vi "Wilt Dryer Cluster Arrays ReadWrite.vi"(0 "Array Label":string(combo)="Aisle1", 1 "Write?":bool, 5 "configuration file path":path=path "C:/data/Wilt Backup.ini", 7 "Array Dryers In":T1[](array[typedef]) {"Night Cycle Count" format="%04d"; "Dryer Details"."Stop Dryer" items=["NO", "YES"]; "Dryer Details"."24 Hour Water Injection" items=["NO", "YES"]; "Dryer Details"."Run w/o Newfi" items=["NO", "YES"]; "Day Cycle Count" format="%04d"}, 11 "error in (no error)":errorcluster) -> (8 "Array Dryers Out":T1[](array[typedef]) {"Night Cycle Count" format="%04d"; "Dryer Details"."Stop Dryer" items=["NO", "YES"]; "Dryer Details"."24 Hour Water Injection" items=["NO", "YES"]; "Dryer Details"."Run w/o Newfi" items=["NO", "YES"]; "Day Cycle Count" format="%04d"}, 15 "error out":errorcluster)   [LabVIEW 2012]
uses:
  <vilib>/Utility/VariantDataType/Type.ctl
  Dryer.ctl
  Dryer Details.ctl
  <vilib>/Utility/config.llb/Write Key (Double).vi
  <vilib>/Utility/config.llb/Write Key (String).vi
  <vilib>/Utility/config.llb/Write Key (Path).vi
  <vilib>/Utility/config.llb/Write Key (I32).vi
  <vilib>/Utility/config.llb/Write Key (U32).vi
  <vilib>/Utility/config.llb/Write Key (Boolean).vi
  <vilib>/Utility/config.llb/Read Key (Double).vi
  <vilib>/Utility/config.llb/Read Key (String).vi
  <vilib>/Utility/config.llb/Read Key (Path).vi
  <vilib>/Utility/config.llb/Read Key (I32).vi
  <vilib>/Utility/config.llb/Read Key (U32).vi
  <vilib>/Utility/config.llb/Read Key (Boolean).vi
  <vilib>/Utility/config.llb/NI_LVConfig.lvlib
  <vilib>/Utility/VariantDataType/VariantType.lvlib
panel:
  out "Label.Text 2":string
  out "Local Control?":bool
  in  "Array Dryers Display":T1[](array[typedef]) {"Night Cycle Count" format="%04d"; "Dryer Details"."Stop Dryer" items=["NO", "YES"]; "Dryer Details"."24 Hour Water Injection" items=["NO", "YES"]; "Dryer Details"."Run w/o Newfi" items=["NO", "YES"]; "Day Cycle Count" format="%04d"}
  out "value":string
  in  "Dryer Variable":T1 {"Night Cycle Count" format="%04d"; "Dryer Details"."Stop Dryer" items=["NO", "YES"]; "Dryer Details"."24 Hour Water Injection" items=["NO", "YES"]; "Dryer Details"."Run w/o Newfi" items=["NO", "YES"]; "Day Cycle Count" format="%04d"}
  out "String array out":string="[1,23-2-3]\n[4-3,22-2]\n[3-4,01-8]\n[0-7-6,66]"
  out "Label.Text":string
  out "Type Enum":T3
  # "D"
  # "N"
  # "D"
  # "N"
  # "D"
  # "N"
  # "D"
  # "N"
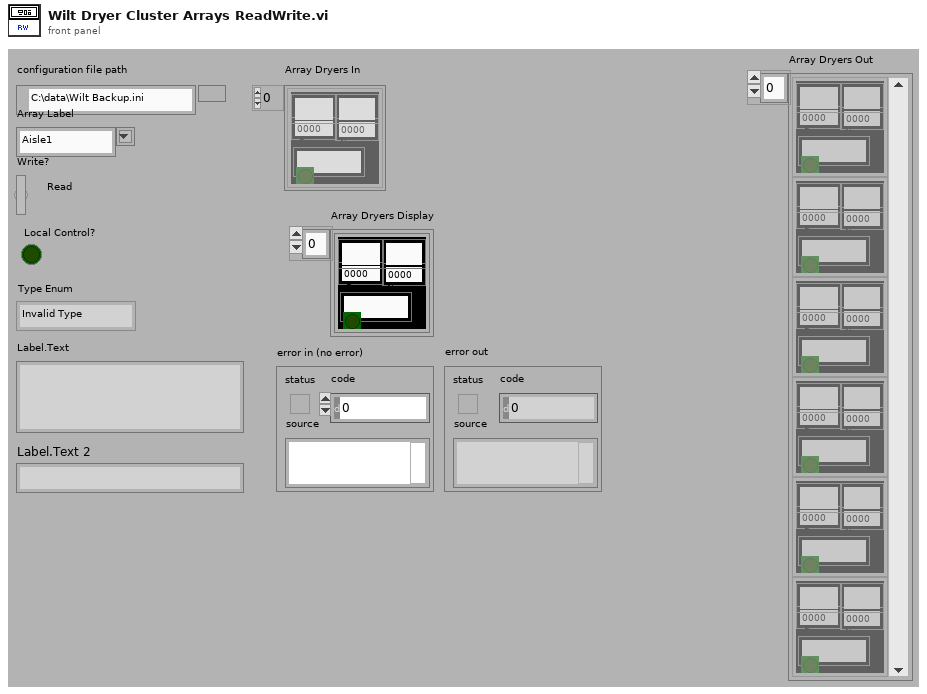
[diagram p1: front panel]
types:
  T1 = typedef "Dryer.ctl" = cluster{"Lab ID":string, "Day Cycle Count":i32, "Station Label":string, "Dryer Details":T2, "Sample Record ":string[], "Hist Record ":string[][], "Status Color":u32, "Boolean":bool, "Com Port":u8, "Bad Com Count":i32, "Current Run Start Time":dbl, "Night Cycle Count":i32, "Station Index":i32, "Cycle Index":string, "Audit Alert":bool}
  T2 = typedef "Dryer Details.ctl" = cluster{"Station":string, "Cycle Count Day":string, "Status":string, "Debug ASCII":string, "Notes":string, "Lab ID":string, "Total Time On":string, "TR Number":string, "Cycle Count Night":string, "Time On Day":string, "Time On Night":string, "Run w/o Newfi":i32, "24 Hour Water Injection":i32, "Stop Dryer":i32}
  T3 = typedef "VariantType.lvlib/Type.ctl" = enum8{"Invalid Type", "Void", "I8", "I16", "I32", "I64", "U8", "U16", "U32", "U64", "Single Float", "Double Float", "Extended Float", "Single Complex", "Double Complex", "Extended Complex", "Enum U8", "Enum U16", "Enum U32", "Enum U64", "Single Float With Unit", "Double Float With Unit", "Extended Float With Unit", "Single Complex with Unit", "Double Complex with Unit", "Extended Complex with Unit", "Boolean", "String", "Path", "Picture", "Tag", "Array", "Cluster", "Variant", "LV Variant", "Waveform", "Timestamp", "Digital Waveform", "Digital Data", "ExpressData", "Refnum", "External Data", "VI", "Poly VI", "LabVIEW Class Instance", "Fixed Point"}
  T4 = typedef "NI_LVConfig.lvlib/Config Data RefNum.ctl" = refnum<k1>
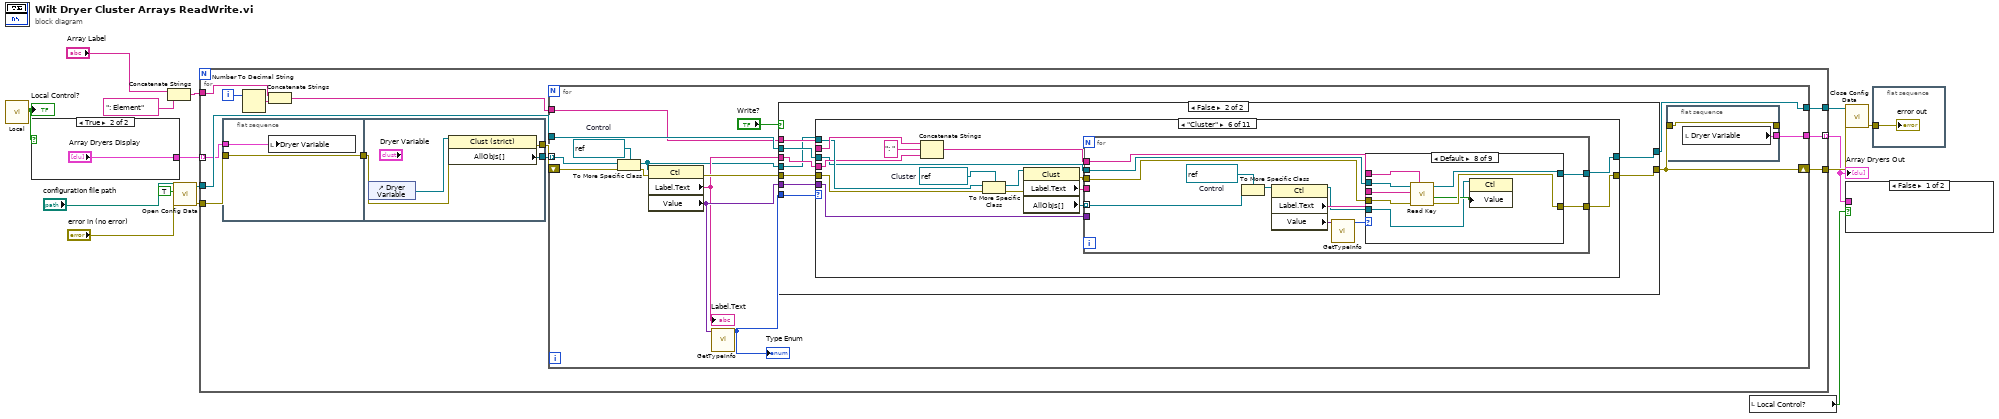
[diagram p0: block diagram]
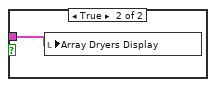
[diagram p2: hidden frame]
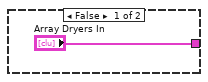
[diagram p3: hidden frame]
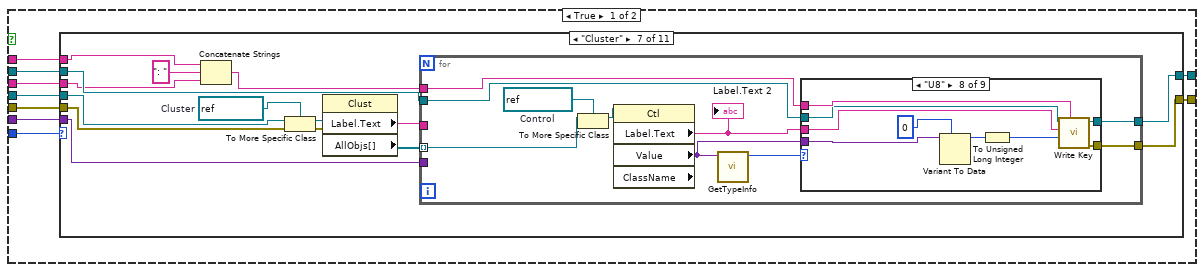
[diagram p4: hidden frame]
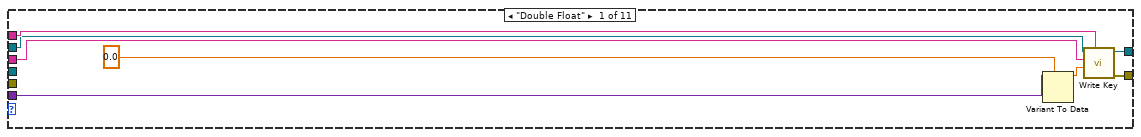
[diagram p5: hidden frame]
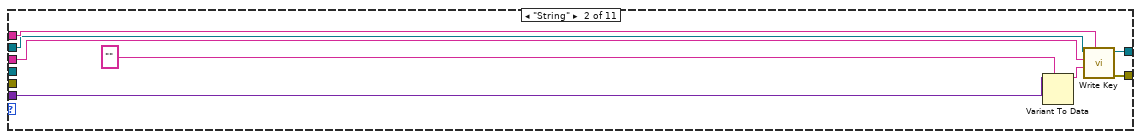
[diagram p6: hidden frame]
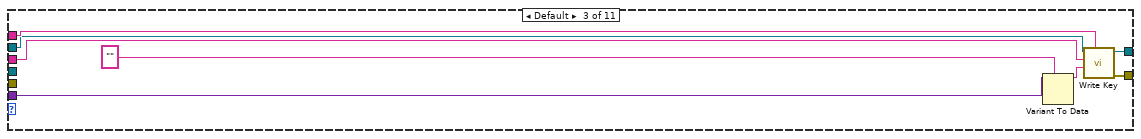
[diagram p7: hidden frame]
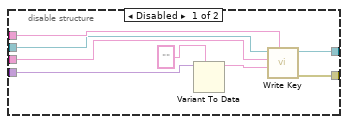
[diagram p9: hidden frame]
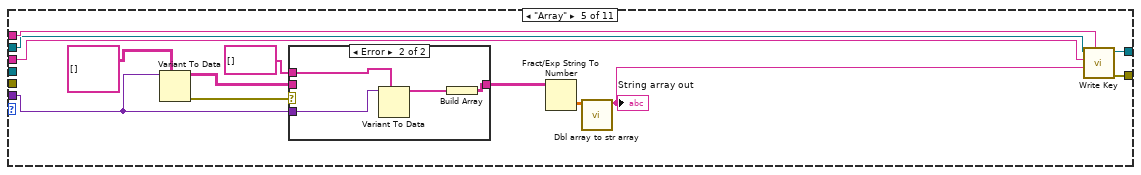
[diagram p10: hidden frame]
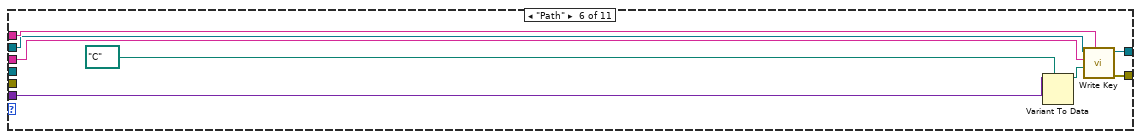
[diagram p12: hidden frame]
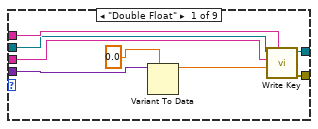
[diagram p13: hidden frame]
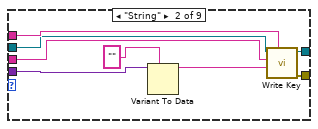
[diagram p14: hidden frame]
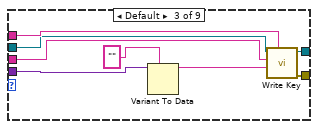
[diagram p15: hidden frame]
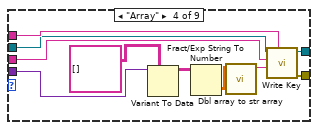
[diagram p16: hidden frame]
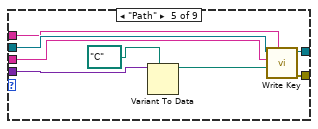
[diagram p17: hidden frame]
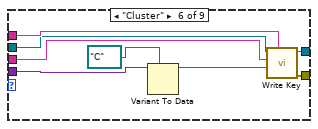
[diagram p18: hidden frame]
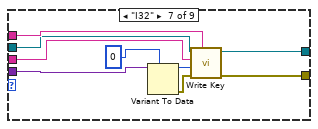
[diagram p19: hidden frame]
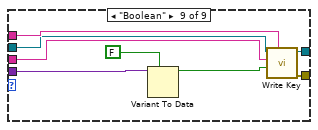
[diagram p20: hidden frame]
diagram:
  n1 = call "Local.vi"() -> ("Local?"=w1:bool)  [unwired: 11 in]
  "Local Control?" <- w1
  n2 = case shown="True" w1 {
    tunnel: ["Array Dryers In" "Array Dryers Display"] -> w3
    frame False {
    }
    frame True {
    }
  }
  n3 = Concatenate Strings("Array Label", ": Element" ("string")) -> (w8:string)
  n4 = call <vilib>:"Open Config Data.vi"("error in (no error)"="error in (no error)", "create file if necessary (T)"=TRUE, "configuration file path"="configuration file path") -> ("error out"=w11:errorcluster, "refnum"=w13:T4)  [unwired: 6 in, 1 out]
  n5 = for {
    tunnel: w11 -> [w29]
    tunnel: w3 -> [w25] mode=indexing
    tunnel: w13 -> [w27]
    tunnel: w8 -> [w23]
    tunnel: [w20] -> w6
    tunnel: [w19] -> w5
    tunnel: [w18] -> w4 mode=indexing
    i -> [w21]
    n6 = flat-sequence {
      tunnel: w29 -> [w32]
      tunnel: [w32] -> w26
      tunnel: w25 -> [w31]
      tunnel: [w36] -> w30
      tunnel: [w34] -> w28
      tunnel: w26 -> [w35]
      frame #0 {
        n7 = local write "Dryer Variable"(w31) -> ()
      }
      frame #1 {
        n8 = control-ref of="Dryer Variable"() -> (w33:refnum<vi>)
        n9 = property class="Clust (strict)"(reference=w33, error in=w35) -> (error out=w34:errorcluster, "AllObjs[]"=w36:refnum<vi>[])  [unwired: 1 out]
      }
    }
    n10 = Number To Decimal String(number=w21) -> (decimal integer string=w24:string)  [unwired: 1 in]
    n11 = Concatenate Strings(w23, w24) -> (w22:string)
    n12 = for {
      tunnel: w30 -> [w51] mode=indexing
      tunnel: w27 -> [w49]
      tunnel: [w48] -> w19
      shift-right: [w39] -> w20
      shift-left: w28 -> [w47]
      tunnel: w22 -> [w40]
      tunnel: [w38] -> w18
      w50 = refnum<vi> refnum  # Control
      n13 = To More Specific Class(target class=w50, reference=w51, error in=w47) -> (specific class reference=w37:refnum<vi>, error out=w42:errorcluster)
      n14 = property class="Ctl"(reference=w37, error in=w42) -> (error out=w43:errorcluster, "Label.Text"=w41:string, "Value"=w44:variant)  [unwired: 1 out]
      "Label.Text" <- w41
      n15 = call <vilib>:"GetTypeInfo.vi"("Variant"=w44) -> ("Type Enum"=w45:T3)  [unwired: 6 in, 4 out]
      "Type Enum" <- w45
      n16 = case shown="False" "Write?" {
        tunnel: w40 -> [w62 w269]
        tunnel: w41 -> [w61 w268]
        tunnel: w44 -> [w60 w261]
        tunnel: w49 -> [w59 w267]
        tunnel: [w58 w266] -> w39
        tunnel: [w57 w265] -> w48
        tunnel: w37 -> [w54 w264]
        tunnel: w45 -> [w56 w263]
        tunnel: w43 -> [w55 w262]
        frame True {
          n17 = case shown="\"Cluster\"" w56 {
            tunnel: w62 -> [w70 w78 w86 w92 w113 w126 w129 w235 w243 w252 w260]
            tunnel: w61 -> [w69 w77 w85 w91 w112 w125 w128 w234 w242 w251 w259]
            tunnel: w60 -> [w68 w76 w84 w90 w102 w124 w137 w233 w241 w250 w258]
            tunnel: w59 -> [w67 w75 w83 w89 w111 w123 w131 w232 w240 w249 w257]
            tunnel: [w66 w74 w82 w88 w110 w122 w135 w231 w239 w248 w256] -> w58
            tunnel: [w65 w73 w81 w87 w109 w121 w136 w230 w238 w247 w255] -> w57
            tunnel: w55 -> [_ _ _ _ _ _ w138 _ _ _ _]
            tunnel: w54 -> [_ _ _ _ _ _ w133 _ _ _ _]
            frame "Double Float" {
              n18 = Variant To Data(type=0.0, Variant=w68) -> (data=w64:dbl)  [unwired: 1 in, 1 out]
              n19 = call-poly <vilib>:"Write Key.vi"("section"=w70, "value"=w64, "key"=w69, "refnum"=w67) -> ("error out"=w66:errorcluster, "refnum out"=w65:T4)  [unwired: 5 in, 1 out]
            }
            frame "String" {
              n20 = Variant To Data(type="" ("Label.Text"), Variant=w76) -> (data=w72:string)  [unwired: 1 in, 1 out]
              n21 = call-poly <vilib>:"Write Key.vi"("section"=w78, "value"=w72, "key"=w77, "refnum"=w75) -> ("error out"=w74:errorcluster, "refnum out"=w73:T4)  [unwired: 5 in, 1 out]
            }
            frame Default {
              n22 = Variant To Data(type="" ("Label.Text"), Variant=w84) -> (data=w80:string)  [unwired: 1 in, 1 out]
              n23 = call-poly <vilib>:"Write Key.vi"("section"=w86, "value"=w80, "key"=w85, "refnum"=w83) -> ("error out"=w82:errorcluster, "refnum out"=w81:T4)  [unwired: 5 in, 1 out]
            }
            frame "Void" {
              n24 = disable-structure shown="Enabled" {
                disable-tunnel: w92 -> [w100 _]
                disable-tunnel: w91 -> [w99 _]
                disable-tunnel: w90 -> [w98 _]
                disable-tunnel: w89 -> [w97 _]
                disable-tunnel: [w96 _] -> w88
                disable-tunnel: [w95 _] -> w87
                frame Disabled {
                  n25 = Variant To Data(type="" ("Label.Text"), Variant=w98) -> (data=w94:string)  [unwired: 1 in, 1 out]
                  n26 = call-poly <vilib>:"Write Key.vi"("section"=w100, "value"=w94, "key"=w99, "refnum"=w97) -> ("error out"=w96:errorcluster, "refnum out"=w95:T4)  [unwired: 5 in, 1 out]
                }
                frame Enabled {
                }
              }
            }
            frame "Array" {
              n27 = Variant To Data(type=string[][] [], Variant=w102) -> (data=w104:string[][], error out=w105:errorcluster)  [unwired: 1 in]
              n28 = case shown="Error" w105 {
                tunnel: [w114 w115] -> w103
                tunnel: w104 -> [w114 _]
                tunnel: w102 -> [_ w118]
                tunnel: string[] [] -> [_ w117]
                frame No Error {
                }
                frame Error {
                  n29 = Variant To Data(type=w117, Variant=w118) -> (data=w116:string[])  [unwired: 1 in, 1 out]
                  n30 = Build Array(w116) -> (w115:string[][])
                }
              }
              n31 = Fract/Exp String To Number(string=w103) -> (number=w107:dbl[][])  [unwired: 3 in, 1 out]
              n32 = call "Dbl array to str array.vi"("Array in"=w107) -> ("String array out"=w106:string)  [unwired: 9 in, 1 out]
              "String array out" <- w106
              n33 = call-poly <vilib>:"Write Key.vi"("section"=w113, "value"=w106, "key"=w112, "refnum"=w111) -> ("error out"=w110:errorcluster, "refnum out"=w109:T4)  [unwired: 5 in, 1 out]
            }
            frame "Path" {
              n34 = Variant To Data(type=path "C:/" ("configuration file path 2"), Variant=w124) -> (data=w120:path)  [unwired: 1 in, 1 out]
              n35 = call-poly <vilib>:"Write Key.vi"("section"=w126, "value"=w120, "key"=w125, "refnum"=w123) -> ("error out"=w122:errorcluster, "refnum out"=w121:T4)  [unwired: 5 in, 1 out]
            }
            frame "Cluster" {
              w141 = refnum<vi> refnum  # Cluster
              n36 = Concatenate Strings(w129, ": " ("string"), w128) -> (w130:string)
              n37 = To More Specific Class(target class=w141, reference=w133, error in=w138) -> (specific class reference=w140:refnum<vi>, error out=w139:errorcluster)
              n38 = property class="Clust"(reference=w140, error in=w139) -> ("Label.Text"=w134:string, "AllObjs[]"=w132:refnum<vi>[])  [unwired: 2 out]
              n39 = for {
                tunnel: w137 -> [_]
                tunnel: w130 -> [w151]
                tunnel: w132 -> [w146] mode=indexing
                tunnel: [w150] -> w136
                tunnel: [w149] -> w135
                tunnel: w134 -> [_]
                tunnel: w131 -> [w145]
                w148 = refnum<vi> refnum  # Control
                n40 = To More Specific Class(target class=w148, reference=w146) -> (specific class reference=w147:refnum<vi>)  [unwired: 1 in, 1 out]
                n41 = property class="Ctl" props=["Label", "Text", "Value", "ClassName"](reference=w147) -> ("Label.Text"=w142:string, "Value"=w143:variant)  [unwired: 1 in, 3 out]
                "Label.Text 2" <- w142
                n42 = call <vilib>:"GetTypeInfo.vi"("Variant"=w143) -> ("Type Enum"=w144:T3)  [unwired: 6 in, 4 out]
                n43 = case shown="\"U8\"" w144 {
                  tunnel: w151 -> [w159 w167 w175 w185 w187 w201 w210 w219 w227]
                  tunnel: w142 -> [w158 w166 w168 w184 w186 w200 w209 w218 w226]
                  tunnel: w143 -> [w157 w165 w174 w183 w193 w199 w208 w217 w225]
                  tunnel: w145 -> [w152 w160 w169 w176 w188 w194 w202 w211 w220]
                  tunnel: [w156 w164 w173 w182 w192 w198 w207 w216 w224] -> w149
                  tunnel: [w155 w163 w172 w181 w191 w197 w206 w215 w223] -> w150
                  frame "Double Float" {
                    n44 = Variant To Data(type=0.0, Variant=w157) -> (data=w153:dbl)  [unwired: 1 in, 1 out]
                    n45 = call-poly <vilib>:"Write Key.vi"("section"=w159, "value"=w153, "key"=w158, "refnum"=w152) -> ("error out"=w156:errorcluster, "refnum out"=w155:T4)  [unwired: 5 in, 1 out]
                  }
                  frame "String" {
                    n46 = Variant To Data(type="" ("Label.Text"), Variant=w165) -> (data=w161:string)  [unwired: 1 in, 1 out]
                    n47 = call-poly <vilib>:"Write Key.vi"("section"=w167, "value"=w161, "key"=w166, "refnum"=w160) -> ("error out"=w164:errorcluster, "refnum out"=w163:T4)  [unwired: 5 in, 1 out]
                  }
                  frame Default {
                    n48 = Variant To Data(type="" ("Label.Text"), Variant=w174) -> (data=w170:string)  [unwired: 1 in, 1 out]
                    n49 = call-poly <vilib>:"Write Key.vi"("section"=w175, "value"=w170, "key"=w168, "refnum"=w169) -> ("error out"=w173:errorcluster, "refnum out"=w172:T4)  [unwired: 5 in, 1 out]
                  }
                  frame "Array" {
                    n50 = Variant To Data(type=string[][] [], Variant=w183) -> (data=w179:string[][])  [unwired: 1 in, 1 out]
                    n51 = Fract/Exp String To Number(string=w179) -> (number=w178:dbl[][])  [unwired: 3 in, 1 out]
                    n52 = call "Dbl array to str array.vi"("Array in"=w178) -> ("String array out"=w177:string)  [unwired: 9 in, 1 out]
                    n53 = call-poly <vilib>:"Write Key.vi"("section"=w185, "value"=w177, "key"=w184, "refnum"=w176) -> ("error out"=w182:errorcluster, "refnum out"=w181:T4)  [unwired: 5 in, 1 out]
                  }
                  frame "Path" {
                    n54 = Variant To Data(type=path "C:/" ("configuration file path 2"), Variant=w193) -> (data=w189:path)  [unwired: 1 in, 1 out]
                    n55 = call-poly <vilib>:"Write Key.vi"("section"=w187, "value"=w189, "key"=w186, "refnum"=w188) -> ("error out"=w192:errorcluster, "refnum out"=w191:T4)  [unwired: 5 in, 1 out]
                  }
                  frame "Cluster" {
                    n56 = Variant To Data(type=path "C:/" ("configuration file path 2"), Variant=w199) -> (data=w195:path)  [unwired: 1 in, 1 out]
                    n57 = call-poly <vilib>:"Write Key.vi"("section"=w201, "value"=w195, "key"=w200, "refnum"=w194) -> ("error out"=w198:errorcluster, "refnum out"=w197:T4)  [unwired: 5 in, 1 out]
                  }
                  frame "I32" {
                    n58 = Variant To Data(type=0, Variant=w208) -> (data=w203:i32, error out=w204:errorcluster)  [unwired: 1 in]
                    n59 = call-poly <vilib>:"Write Key.vi"("section"=w210, "error in (no error)"=w204, "value"=w203, "key"=w209, "refnum"=w202) -> ("error out"=w207:errorcluster, "refnum out"=w206:T4)  [unwired: 4 in, 1 out]
                  }
                  frame "U8" {
                    n60 = Variant To Data(type=u8 0, Variant=w217) -> (data=w214:u8)  [unwired: 1 in, 1 out]
                    n61 = To Unsigned Long Integer(number=w214) -> (unsigned 32bit integer=w212:u32)
                    n62 = call-poly <vilib>:"Write Key.vi"("section"=w219, "value"=w212, "key"=w218, "refnum"=w211) -> ("error out"=w216:errorcluster, "refnum out"=w215:T4)  [unwired: 5 in, 1 out]
                  }
                  frame "Boolean" {
                    n63 = Variant To Data(type=FALSE ("Write? 2"), Variant=w225) -> (data=w222:bool)  [unwired: 1 in, 1 out]
                    n64 = call-poly <vilib>:"Write Key.vi"("section"=w227, "value"=w222, "key"=w226, "refnum"=w220) -> ("error out"=w224:errorcluster, "refnum out"=w223:T4)  [unwired: 5 in, 1 out]
                  }
                }
              }
            }
            frame "I32" {
              n65 = Variant To Data(type=0, Variant=w233) -> (data=w229:i32)  [unwired: 1 in, 1 out]
              n66 = call-poly <vilib>:"Write Key.vi"("section"=w235, "value"=w229, "key"=w234, "refnum"=w232) -> ("error out"=w231:errorcluster, "refnum out"=w230:T4)  [unwired: 5 in, 1 out]
            }
            frame "U32" {
              n67 = Variant To Data(type=0, Variant=w241) -> (data=w237:i32)  [unwired: 1 in, 1 out]
              n68 = call-poly <vilib>:"Write Key.vi"("section"=w243, "value"=w237, "key"=w242, "refnum"=w240) -> ("error out"=w239:errorcluster, "refnum out"=w238:T4)  [unwired: 5 in, 1 out]
            }
            frame "U8" {
              n69 = Variant To Data(type=u8 0, Variant=w250) -> (data=w246:u8)  [unwired: 1 in, 1 out]
              n70 = To Unsigned Long Integer(number=w246) -> (unsigned 32bit integer=w244:u32)
              n71 = call-poly <vilib>:"Write Key.vi"("section"=w252, "value"=w244, "key"=w251, "refnum"=w249) -> ("error out"=w248:errorcluster, "refnum out"=w247:T4)  [unwired: 5 in, 1 out]
            }
            frame "Boolean" {
              n72 = Variant To Data(type=FALSE ("Write? 2"), Variant=w258) -> (data=w254:bool)  [unwired: 1 in, 1 out]
              n73 = call-poly <vilib>:"Write Key.vi"("section"=w260, "value"=w254, "key"=w259, "refnum"=w257) -> ("error out"=w256:errorcluster, "refnum out"=w255:T4)  [unwired: 5 in, 1 out]
            }
          }
        }
        frame False {
          n74 = case shown="\"Cluster\"" w263 {
            tunnel: w269 -> [w276 w292 w300 w311 w319 w335 w428 w436 w444 w452 w460]
            tunnel: w268 -> [w275 w291 w299 w310 w326 w331 w435 w443 w451 w459 w467]
            tunnel: w267 -> [w274 w290 w298 w309 w325 w330 w434 w442 w450 w458 w466]
            tunnel: [w273 w289 w297 w308 w324 w328 w433 w441 w449 w457 w465] -> w266
            tunnel: [w272 w288 w296 w307 w323 w329 w432 w440 w448 w456 w464] -> w265
            tunnel: w264 -> [w271 w286 w294 w302 w321 w332 w430 w438 w446 w454 w462]
            tunnel: w262 -> [w270 w285 w293 w306 w320 w333 w429 w437 w445 w453 w461]
            tunnel: w261 -> [_ _ _ _ _ w334 _ _ _ _ _]
            frame "Void" {
              n75 = disable-structure shown="Enabled" {
                disable-tunnel: w276 -> [w284 _]
                disable-tunnel: w275 -> [w283 _]
                disable-tunnel: w274 -> [w282 _]
                disable-tunnel: [w281 _] -> w273
                disable-tunnel: [w280 _] -> w272
                disable-tunnel: w271 -> [w278 _]
                disable-tunnel: w270 -> [w277 _]
                frame Disabled {
                  n76 = call-poly <vilib>:"Read Key.vi"("section"=w284, "error in (no error)"=w277, "key"=w283, "refnum"=w282) -> ("error out"=w281:errorcluster, "value"=w279:bool, "refnum out"=w280:T4)  [unwired: 4 in, 1 out]
                  n77 = property class="Ctl"(reference=w278, "Value"=w279) -> ()  [unwired: 1 in, 2 out]
                }
                frame Enabled {
                }
              }
            }
            frame "Double Float" {
              n78 = call-poly <vilib>:"Read Key.vi"("section"=w292, "error in (no error)"=w285, "key"=w291, "refnum"=w290) -> ("error out"=w289:errorcluster, "value"=w287:dbl, "refnum out"=w288:T4)  [unwired: 4 in, 1 out]
              n79 = property class="Ctl"(reference=w286, "Value"=w287) -> ()  [unwired: 1 in, 2 out]
            }
            frame "String" {
              n80 = call-poly <vilib>:"Read Key.vi"("section"=w300, "error in (no error)"=w293, "key"=w299, "refnum"=w298) -> ("error out"=w297:errorcluster, "value"=w295:string, "refnum out"=w296:T4)  [unwired: 4 in, 1 out]
              n81 = property class="Ctl"(reference=w294, "Value"=w295) -> ()  [unwired: 1 in, 2 out]
            }
            frame "Array" {
              n82 = call-poly <vilib>:"Read Key.vi"("section"=w311, "error in (no error)"=w306, "key"=w310, "refnum"=w309) -> ("error out"=w308:errorcluster, "value"=w305:string, "refnum out"=w307:T4)  [unwired: 4 in, 1 out]
              "value" <- w305
              n83 = call "Str array to dbl array.vi"("String array in"=w305) -> ("Double array out"=w304:dbl[][])  [unwired: 9 in, 1 out]
              n84 = Number To Fractional String(number=w304) -> (F-format string=w301:string[][])  [unwired: 3 in]
              n85 = property class="Ctl"(reference=w302, "Value"=w301) -> (error out=w303:errorcluster)  [unwired: 1 in, 1 out]
              n86 = case shown="Error" w303 {
                tunnel: w302 -> [_ w318]
                tunnel: w301 -> [_ w317]
                frame No Error {
                }
                frame Error {
                  n87 = Array Subset(array=w317, index (row)=0 ("index")) -> (w314:string[][])  [unwired: 3 in]
                  n88 = Array Size(array=w314) -> (size(s)=w313:i32[])
                  n89 = Multiply Array Elements(1:w313) -> (0:w312:i32)
                  n90 = Reshape Array(w314, w312) -> (w315:string[])
                  n91 = property class="Ctl"(reference=w318, "Value"=w315) -> ()  [unwired: 1 in, 2 out]
                }
              }
            }
            frame "Path" {
              n92 = call-poly <vilib>:"Read Key.vi"("section"=w319, "error in (no error)"=w320, "key"=w326, "refnum"=w325) -> ("error out"=w324:errorcluster, "value"=w322:path, "refnum out"=w323:T4)  [unwired: 4 in, 1 out]
              n93 = property class="Ctl"(reference=w321, "Value"=w322) -> ()  [unwired: 1 in, 2 out]
            }
            frame "Cluster" {
              w342 = refnum<vi> refnum  # Cluster
              n94 = Concatenate Strings(w335, ": " ("string"), w331) -> (w337:string)
              n95 = To More Specific Class(target class=w342, reference=w332, error in=w333) -> (specific class reference=w341:refnum<vi>, error out=w340:errorcluster)
              n96 = property class="Clust"(reference=w341, error in=w340) -> (error out=w327:errorcluster, "Label.Text"=w339:string, "AllObjs[]"=w338:refnum<vi>[])  [unwired: 1 out]
              n97 = for {
                tunnel: w334 -> [_]
                tunnel: w337 -> [w345]
                tunnel: w338 -> [w352] mode=indexing
                tunnel: [w344] -> w329
                tunnel: [w348] -> w328
                tunnel: w339 -> [_]
                tunnel: w330 -> [w347]
                tunnel: w327 -> [w349]
                w354 = refnum<vi> refnum  # Control
                n98 = To More Specific Class(target class=w354, reference=w352) -> (specific class reference=w353:refnum<vi>)  [unwired: 1 in, 1 out]
                n99 = property class="Ctl"(reference=w353) -> (reference out=w346:refnum<vi>, "Label.Text"=w350:string, "Value"=w351:variant)  [unwired: 1 in, 1 out]
                n100 = call <vilib>:"GetTypeInfo.vi"("Variant"=w351) -> ("Type Enum"=w343:T3)  [unwired: 6 in, 4 out]
                n101 = case shown="Default" w343 {
                  tunnel: w345 -> [w362 w370 w378 w387 w388 w396 w404 w412 w420]
                  tunnel: w350 -> [w361 w369 w377 w386 w395 w403 w411 w419 w427]
                  tunnel: w347 -> [w360 w368 w376 w385 w394 w402 w410 w418 w426]
                  tunnel: [w359 w367 w375 w384 w393 w401 w409 w417 w425] -> w348
                  tunnel: [w358 w366 w374 w383 w392 w400 w408 w416 w424] -> w344
                  tunnel: w346 -> [w356 w364 w372 w382 w390 w398 w406 w414 w422]
                  tunnel: w349 -> [w355 w363 w371 w381 w389 w397 w405 w413 w421]
                  frame "Void" {
                    n102 = call-poly <vilib>:"Read Key.vi"("section"=w362, "error in (no error)"=w355, "key"=w361, "refnum"=w360) -> ("error out"=w359:errorcluster, "value"=w357:string, "refnum out"=w358:T4)  [unwired: 4 in, 1 out]
                    n103 = property class="Ctl"(reference=w356, "Value"=w357) -> ()  [unwired: 1 in, 2 out]
                  }
                  frame "Double Float" {
                    n104 = call-poly <vilib>:"Read Key.vi"("section"=w370, "error in (no error)"=w363, "key"=w369, "refnum"=w368) -> ("error out"=w367:errorcluster, "value"=w365:dbl, "refnum out"=w366:T4)  [unwired: 4 in, 1 out]
                    n105 = property class="Ctl"(reference=w364, "Value"=w365) -> ()  [unwired: 1 in, 2 out]
                  }
                  frame "String" {
                    n106 = call-poly <vilib>:"Read Key.vi"("section"=w378, "error in (no error)"=w371, "key"=w377, "refnum"=w376) -> ("error out"=w375:errorcluster, "value"=w373:string, "refnum out"=w374:T4)  [unwired: 4 in, 1 out]
                    n107 = property class="Ctl"(reference=w372, "Value"=w373) -> ()  [unwired: 1 in, 2 out]
                  }
                  frame "Array" {
                    n108 = call-poly <vilib>:"Read Key.vi"("section"=w387, "error in (no error)"=w381, "key"=w386, "refnum"=w385) -> ("error out"=w384:errorcluster, "value"=w380:string, "refnum out"=w383:T4)  [unwired: 4 in, 1 out]
                    n109 = call "Str array to dbl array.vi"("String array in"=w380) -> ("Double array out"=w379:dbl[][])  [unwired: 9 in, 1 out]
                    n110 = property class="Ctl"(reference=w382, "Value"=w379) -> ()  [unwired: 1 in, 2 out]
                  }
                  frame "Path" {
                    n111 = call-poly <vilib>:"Read Key.vi"("section"=w388, "error in (no error)"=w389, "key"=w395, "refnum"=w394) -> ("error out"=w393:errorcluster, "value"=w391:path, "refnum out"=w392:T4)  [unwired: 4 in, 1 out]
                    n112 = property class="Ctl"(reference=w390, "Value"=w391) -> ()  [unwired: 1 in, 2 out]
                  }
                  frame "I32" {
                    n113 = call-poly <vilib>:"Read Key.vi"("section"=w396, "error in (no error)"=w397, "key"=w403, "refnum"=w402) -> ("error out"=w401:errorcluster, "value"=w399:i32, "refnum out"=w400:T4)  [unwired: 4 in, 1 out]
                    n114 = property class="Ctl"(reference=w398, "Value"=w399) -> ()  [unwired: 1 in, 2 out]
                  }
                  frame "U32" {
                    n115 = call-poly <vilib>:"Read Key.vi"("section"=w404, "error in (no error)"=w405, "key"=w411, "refnum"=w410) -> ("error out"=w409:errorcluster, "value"=w407:u32, "refnum out"=w408:T4)  [unwired: 4 in, 1 out]
                    n116 = property class="Ctl"(reference=w406, "Value"=w407) -> ()  [unwired: 1 in, 2 out]
                  }
                  frame Default {
                    n117 = call-poly <vilib>:"Read Key.vi"("section"=w412, "error in (no error)"=w413, "key"=w419, "refnum"=w418) -> ("error out"=w417:errorcluster, "value"=w415:bool, "refnum out"=w416:T4)  [unwired: 4 in, 1 out]
                    n118 = property class="Ctl"(reference=w414, "Value"=w415) -> ()  [unwired: 1 in, 2 out]
                  }
                  frame "Boolean" {
                    n119 = call-poly <vilib>:"Read Key.vi"("section"=w420, "error in (no error)"=w421, "key"=w427, "refnum"=w426) -> ("error out"=w425:errorcluster, "value"=w423:bool, "refnum out"=w424:T4)  [unwired: 4 in, 1 out]
                    n120 = property class="Ctl"(reference=w422, "Value"=w423) -> ()  [unwired: 1 in, 2 out]
                  }
                }
              }
            }
            frame "I32" {
              n121 = call-poly <vilib>:"Read Key.vi"("section"=w428, "error in (no error)"=w429, "key"=w435, "refnum"=w434) -> ("error out"=w433:errorcluster, "value"=w431:i32, "refnum out"=w432:T4)  [unwired: 4 in, 1 out]
              n122 = property class="Ctl"(reference=w430, "Value"=w431) -> ()  [unwired: 1 in, 2 out]
            }
            frame "U32" {
              n123 = call-poly <vilib>:"Read Key.vi"("section"=w436, "error in (no error)"=w437, "key"=w443, "refnum"=w442) -> ("error out"=w441:errorcluster, "value"=w439:u32, "refnum out"=w440:T4)  [unwired: 4 in, 1 out]
              n124 = property class="Ctl"(reference=w438, "Value"=w439) -> ()  [unwired: 1 in, 2 out]
            }
            frame "U8" {
              n125 = call-poly <vilib>:"Read Key.vi"("section"=w444, "error in (no error)"=w445, "key"=w451, "refnum"=w450) -> ("error out"=w449:errorcluster, "value"=w447:u32, "refnum out"=w448:T4)  [unwired: 4 in, 1 out]
              n126 = property class="Ctl"(reference=w446, "Value"=w447) -> ()  [unwired: 1 in, 2 out]
            }
            frame Default {
              n127 = call-poly <vilib>:"Read Key.vi"("section"=w452, "error in (no error)"=w453, "key"=w459, "refnum"=w458) -> ("error out"=w457:errorcluster, "value"=w455:string, "refnum out"=w456:T4)  [unwired: 4 in, 1 out]
              n128 = property class="Ctl"(reference=w454, "Value"=w455) -> ()  [unwired: 1 in, 2 out]
            }
            frame "Boolean" {
              n129 = call-poly <vilib>:"Read Key.vi"("section"=w460, "error in (no error)"=w461, "key"=w467, "refnum"=w466) -> ("error out"=w465:errorcluster, "value"=w463:bool, "refnum out"=w464:T4)  [unwired: 4 in, 1 out]
              n130 = property class="Ctl"(reference=w462, "Value"=w463) -> ()  [unwired: 1 in, 2 out]
            }
          }
        }
      }
      n131 = flat-sequence {
        tunnel: [w53] -> _
        tunnel: w39 -> [w53]
        tunnel: [w52] -> w38
        frame #0 {
          n132 = local read "Dryer Variable"() -> (w52:T1)
        }
      }
    }
  }
  "Array Dryers Out" <- w4
  n133 = local read "Local Control?"() -> (w2:bool)
  n134 = call <vilib>:"Close Config Data.vi"("error in (no error)"=w6, "refnum"=w5) -> ("error out"=w7:errorcluster)  [unwired: 8 in, 1 out]
  n135 = case shown="False" w2 {
    tunnel: w4 -> [_ w468]
    frame False {
    }
    frame True {
      n136 = local write "Array Dryers Display"(w468) -> ()
    }
  }
  n137 = flat-sequence {
    tunnel: w7 -> [w469]
    frame #0 {
      "error out" <- w469
    }
  }
